vi "Draw Object Tree.vi"() -> ()   [LabVIEW 2019]
uses:
  Logger_class/ObjData.ctl
  Logger_class/ObjType.ctl
  Logger_class/Logger.lvclass
panel:
  out "All Objects":set{T1}(c389)={{"object_tag"="AI0", "parent_tag"="STAND", "object_type"=enum."AI", "description"="Óðîâåíü  ìàñëà"}, {"object_tag"="AI0.HI", "parent_tag"="AI0", "object_type"=enum."AA", "description"="AI0.HI"}, {"object_tag"="AI0.HIHI", "parent_tag"="AI0", "object_type"=enum."AA", "description"="AI0.HIHI"}, {"object_tag"="AI0.LO", "parent_tag"="AI0", "object_type"=enum."AA", "description"="AI0.LO"}, {"object_tag"="AI0.LOLO", "parent_tag"="AI0", "object_type"=enum."AA", "description"="AI0.LOLO"}, {"object_tag"="AI0.OutOfRangeMax", "parent_tag"="AI0", "object_type"=enum."AA", "description"="AI0.OutOfRangeMax"}, {"object_tag"="AI0.OutOfRangeMin", "parent_tag"="AI0", "object_type"=enum."AA", "description"="AI0.OutOfRangeMin"}, {"object_tag"="AI1", "parent_tag"="STAND", "object_type"=enum."AI", "description"="Óðîâåíü  ìàñëà"}, {"object_tag"="AI1.HI", "parent_tag"="AI1", "object_type"=enum."AA", "description"="AI1.HI"}, {"object_tag"="AI1.HIHI", "parent_tag"="AI1", "object_type"=enum."AA", "description"="AI1.HIHI"}, {"object_tag"="AI1.LO", "parent_tag"="AI1", "object_type"=enum."AA", "description"="AI1.LO"}, {"object_tag"="AI1.LOLO", "parent_tag"="AI1", "object_type"=enum."AA", "description"="AI1.LOLO"}, {"object_tag"="AI1.OutOfRangeMax", "parent_tag"="AI1", "object_type"=enum."AA", "description"="AI1.OutOfRangeMax"}, {"object_tag"="AI1.OutOfRangeMin", "parent_tag"="AI1", "object_type"=enum."AA", "description"="AI1.OutOfRangeMin"}, {"object_tag"="AI10", "parent_tag"="STAND", "object_type"=enum."AI", "description"="Äàò÷èê äàâëåíèÿ â ëèíèè èçìåðåíèÿ óòå÷åê"}, {"object_tag"="AI10.HI", "parent_tag"="AI10", "object_type"=enum."AA", "description"="AI10.HI"}, {"object_tag"="AI10.HIHI", "parent_tag"="AI10", "object_type"=enum."AA", "description"="AI10.HIHI"}, {"object_tag"="AI10.LO", "parent_tag"="AI10", "object_type"=enum."AA", "description"="AI10.LO"}, {"object_tag"="AI10.LOLO", "parent_tag"="AI10", "object_type"=enum."AA", "description"="AI10.LOLO"}, {"object_tag"="AI10.OutOfRangeMax", "parent_tag"="AI10", "object_type"=enum."AA", "description"="AI10.OutOfRangeMax"}, {"object_tag"="AI10.OutOfRangeMin", "parent_tag"="AI10", "object_type"=enum."AA", "description"="AI10.OutOfRangeMin"}, {"object_tag"="AI2", "parent_tag"="STAND", "object_type"=enum."AI", "description"="Òåìïåðàòóðà ìàñëà"}, {"object_tag"="AI2.HI", "parent_tag"="AI2", "object_type"=enum."AA", "description"="AI2.HI"}, {"object_tag"="AI2.HIHI", "parent_tag"="AI2", "object_type"=enum."AA", "description"="AI2.HIHI"}, {"object_tag"="AI2.LO", "parent_tag"="AI2", "object_type"=enum."AA", "description"="AI2.LO"}, {"object_tag"="AI2.LOLO", "parent_tag"="AI2", "object_type"=enum."AA", "description"="AI2.LOLO"}, {"object_tag"="AI2.OutOfRangeMax", "parent_tag"="AI2", "object_type"=enum."AA", "description"="AI2.OutOfRangeMax"}, {"object_tag"="AI2.OutOfRangeMin", "parent_tag"="AI2", "object_type"=enum."AA", "description"="AI2.OutOfRangeMin"}, {"object_tag"="AI3", "parent_tag"="STAND", "object_type"=enum."AI", "description"="Òåìïåðàòóðà ìàñëà"}, {"object_tag"="AI3.HI", "parent_tag"="AI3", "object_type"=enum."AA", "description"="AI3.HI"}, {"object_tag"="AI3.HIHI", "parent_tag"="AI3", "object_type"=enum."AA", "description"="AI3.HIHI"}, {"object_tag"="AI3.LO", "parent_tag"="AI3", "object_type"=enum."AA", "description"="AI3.LO"}, {"object_tag"="AI3.LOLO", "parent_tag"="AI3", "object_type"=enum."AA", "description"="AI3.LOLO"}, {"object_tag"="AI3.OutOfRangeMax", "parent_tag"="AI3", "object_type"=enum."AA", "description"="AI3.OutOfRangeMax"}, {"object_tag"="AI3.OutOfRangeMin", "parent_tag"="AI3", "object_type"=enum."AA", "description"="AI3.OutOfRangeMin"}, {"object_tag"="AI4", "parent_tag"="STAND", "object_type"=enum."AI", "description"="Îáðàòíàÿ ñâÿçü  îò êëàïàíà"}, {"object_tag"="AI4.HI", "parent_tag"="AI4", "object_type"=enum."AA", "description"="AI4.HI"}, {"object_tag"="AI4.HIHI", "parent_tag"="AI4", "object_type"=enum."AA", "description"="AI4.HIHI"}, {"object_tag"="AI4.LO", "parent_tag"="AI4", "object_type"=enum."AA", "description"="AI4.LO"}, {"object_tag"="AI4.LOLO", "parent_tag"="AI4", "object_type"=enum."AA", "description"="AI4.LOLO"}, {"object_tag"="AI4.OutOfRangeMax", "parent_tag"="AI4", "object_type"=enum."AA", "description"="AI4.OutOfRangeMax"}, {"object_tag"="AI4.OutOfRangeMin", "parent_tag"="AI4", "object_type"=enum."AA", "description"="AI4.OutOfRangeMin"}, {"object_tag"="AI5", "parent_tag"="STAND", "object_type"=enum."AI", "description"="äàâëåíèå ïîñëå íàñîñà ÂÄ"}, {"object_tag"="AI5.HI", "parent_tag"="AI5", "object_type"=enum."AA", "description"="AI5.HI"}, {"object_tag"="AI5.HIHI", "parent_tag"="AI5", "object_type"=enum."AA", "description"="AI5.HIHI"}, {"object_tag"="AI5.LO", "parent_tag"="AI5", "object_type"=enum."AA", "description"="AI5.LO"}, {"object_tag"="AI5.LOLO", "parent_tag"="AI5", "object_type"=enum."AA", "description"="AI5.LOLO"}, {"object_tag"="AI5.OutOfRangeMax", "parent_tag"="AI5", "object_type"=enum."AA", "description"="AI5.OutOfRangeMax"}, {"object_tag"="AI5.OutOfRangeMin", "parent_tag"="AI5", "object_type"=enum."AA", "description"="AI5.OutOfRangeMin"}, {"object_tag"="AI6", "parent_tag"="STAND", "object_type"=enum."AI", "description"="Äàâëåíèå â îáðàçöå"}, {"object_tag"="AI6.HI", "parent_tag"="AI6", "object_type"=enum."AA", "description"="AI6.HI"}, {"object_tag"="AI6.HIHI", "parent_tag"="AI6", "object_type"=enum."AA", "description"="AI6.HIHI"}, {"object_tag"="AI6.LO", "parent_tag"="AI6", "object_type"=enum."AA", "description"="AI6.LO"}, {"object_tag"="AI6.LOLO", "parent_tag"="AI6", "object_type"=enum."AA", "description"="AI6.LOLO"}, {"object_tag"="AI6.OutOfRangeMax", "parent_tag"="AI6", "object_type"=enum."AA", "description"="AI6.OutOfRangeMax"}, {"object_tag"="AI6.OutOfRangeMin", "parent_tag"="AI6", "object_type"=enum."AA", "description"="AI6.OutOfRangeMin"}, {"object_tag"="AI7", "parent_tag"="STAND", "object_type"=enum."AI", "description"="Äàâëåíèå â êàìåðå"}, {"object_tag"="AI7.HI", "parent_tag"="AI7", "object_type"=enum."AA", "description"="AI7.HI"}, {"object_tag"="AI7.HIHI", "parent_tag"="AI7", "object_type"=enum."AA", "description"="AI7.HIHI"}, {"object_tag"="AI7.LO", "parent_tag"="AI7", "object_type"=enum."AA", "description"="AI7.LO"}, {"object_tag"="AI7.LOLO", "parent_tag"="AI7", "object_type"=enum."AA", "description"="AI7.LOLO"}, {"object_tag"="AI7.OutOfRangeMax", "parent_tag"="AI7", "object_type"=enum."AA", "description"="AI7.OutOfRangeMax"}, {"object_tag"="AI7.OutOfRangeMin", "parent_tag"="AI7", "object_type"=enum."AA", "description"="AI7.OutOfRangeMin"}, {"object_tag"="AI8", "parent_tag"="STAND", "object_type"=enum."AI", "description"="Äàâëåíèå  â  ëèíèè ïîäà÷è âîçäóõà â  áëîê ÏÏÂ"}, {"object_tag"="AI8.HI", "parent_tag"="AI8", "object_type"=enum."AA", "description"="AI8.HI"}, {"object_tag"="AI8.HIHI", "parent_tag"="AI8", "object_type"=enum."AA", "description"="AI8.HIHI"}, {"object_tag"="AI8.LO", "parent_tag"="AI8", "object_type"=enum."AA", "description"="AI8.LO"}, {"object_tag"="AI8.LOLO", "parent_tag"="AI8", "object_type"=enum."AA", "description"="AI8.LOLO"}, {"object_tag"="AI8.OutOfRangeMax", "parent_tag"="AI8", "object_type"=enum."AA", "description"="AI8.OutOfRangeMax"}, {"object_tag"="AI8.OutOfRangeMin", "parent_tag"="AI8", "object_type"=enum."AA", "description"="AI8.OutOfRangeMin"}, {"object_tag"="AI9", "parent_tag"="STAND", "object_type"=enum."AI", "description"="Äàâëåíèå  â  ëèíèè ïîäà÷è âîçäóõà ïîñëå áëîêà ÏÏÂ"}, {"object_tag"="AI9.HI", "parent_tag"="AI9", "object_type"=enum."AA", "description"="AI9.HI"}, {"object_tag"="AI9.HIHI", "parent_tag"="AI9", "object_type"=enum."AA", "description"="AI9.HIHI"}, {"object_tag"="AI9.LO", "parent_tag"="AI9", "object_type"=enum."AA", "description"="AI9.LO"}, {"object_tag"="AI9.LOLO", "parent_tag"="AI9", "object_type"=enum."AA", "description"="AI9.LOLO"}, {"object_tag"="AI9.OutOfRangeMax", "parent_tag"="AI9", "object_type"=enum."AA", "description"="AI9.OutOfRangeMax"}, {"object_tag"="AI9.OutOfRangeMin", "parent_tag"="AI9", "object_type"=enum."AA", "description"="AI9.OutOfRangeMin"}, {"object_tag"="DI0", "parent_tag"="STAND", "object_type"=enum."DI", "description"="Êîíòàêòîð"}, {"object_tag"="DI1", "parent_tag"="STAND", "object_type"=enum."DI", "description"="Àâòîìàò"}, {"object_tag"="DI10", "parent_tag"="STAND", "object_type"=enum."DI", "description"="QF4"}, {"object_tag"="DI11", "parent_tag"="STAND", "object_type"=enum."DI", "description"="QF5"}, {"object_tag"="DI12", "parent_tag"="STAND", "object_type"=enum."DI", "description"="Êíîïêà ñáðîñà îøèáêè SB1"}, {"object_tag"="DI13", "parent_tag"="STAND", "object_type"=enum."DI", "description"="Êíîïêà çàïóñêà SB2"}, {"object_tag"="DI14", "parent_tag"="STAND", "object_type"=enum."DI", "description"="Êíîïêà îñòàíîâêè SB3"}, {"object_tag"="DI15", "parent_tag"="STAND", "object_type"=enum."DI", "description"="Êíîïêà àâàðèéíîé îñòàíîâêè SB4"}, {"object_tag"="DI16", "parent_tag"="STAND", "object_type"=enum."DI", "description"="Ïåðåêëþ÷àòåëü ðó÷íîå/àâòî SA1"}, {"object_tag"="DI17", "parent_tag"="STAND", "object_type"=enum."DI", "description"="Èñòî÷íèê ïèòàíèÿ 24 Â"}, {"object_tag"="DI18", "parent_tag"="STAND", "object_type"=enum."DI", "description"="DI 18"}, {"object_tag"="DI19", "parent_tag"="STAND", "object_type"=enum."DI", "description"="DI 19"}, {"object_tag"="DI2", "parent_tag"="STAND", "object_type"=enum."DI", "description"="Êîíòàêòîð"}, {"object_tag"="DI20", "parent_tag"="STAND", "object_type"=enum."DI", "description"="DI 20"}, {"object_tag"="DI21", "parent_tag"="STAND", "object_type"=enum."DI", "description"="DI 21"}, {"object_tag"="DI22", "parent_tag"="STAND", "object_type"=enum."DI", "description"="DI 22"}, {"object_tag"="DI23", "parent_tag"="STAND", "object_type"=enum."DI", "description"="DI 23"}, {"object_tag"="DI24", "parent_tag"="STAND", "object_type"=enum."DI", "description"="DI 24"}, {"object_tag"="DI25", "parent_tag"="STAND", "object_type"=enum."DI", "description"="DI 25"}, {"object_tag"="DI26", "parent_tag"="STAND", "object_type"=enum."DI", "description"="DI 26"}, {"object_tag"="DI27", "parent_tag"="STAND", "object_type"=enum."DI", "description"="DI 27"}, {"object_tag"="DI28", "parent_tag"="STAND", "object_type"=enum."DI", "description"="DI 28"}, {"object_tag"="DI29", "parent_tag"="STAND", "object_type"=enum."DI", "description"="DI 29"}, {"object_tag"="DI3", "parent_tag"="STAND", "object_type"=enum."DI", "description"="Àâòîìàò"}, {"object_tag"="DI30", "parent_tag"="STAND", "object_type"=enum."DI", "description"="DI 30"}, {"object_tag"="DI31", "parent_tag"="STAND", "object_type"=enum."DI", "description"="DI 31"}, {"object_tag"="DI4", "parent_tag"="STAND", "object_type"=enum."DI", "description"="Êîíòàêòîð"}, {"object_tag"="DI5", "parent_tag"="STAND", "object_type"=enum."DI", "description"="Àâòîìàò"}, {"object_tag"="DI6", "parent_tag"="STAND", "object_type"=enum."DI", "description"="QF1"}, {"object_tag"="DI7", "parent_tag"="STAND", "object_type"=enum."DI", "description"="QF2"}, {"object_tag"="DI8", "parent_tag"="STAND", "object_type"=enum."DI", "description"="QF3"}, {"object_tag"="DI9", "parent_tag"="STAND", "object_type"=enum."DI", "description"="Ðåëå êîíòðîëÿ ôàç"}, {"object_tag"="M12", "parent_tag"="PMG", "object_type"=enum."Device", "description"="M12"}, {"object_tag"="M12.Contactor Error", "parent_tag"="M12", "object_type"=enum."DA", "description"=""}, {"object_tag"="M12.OFF_Error", "parent_tag"="M12", "object_type"=enum."DA", "description"=""}, {"object_tag"="M12.ON_Error", "parent_tag"="M12", "object_type"=enum."DA", "description"=""}, {"object_tag"="M12.UnOFF_Error", "parent_tag"="M12", "object_type"=enum."DA", "description"=""}, {"object_tag"="M12.UnON_Error", "parent_tag"="M12", "object_type"=enum."DA", "description"=""}, {"object_tag"="M21", "parent_tag"="PMG", "object_type"=enum."Device", "description"="M21"}, {"object_tag"="M21.Contactor Error", "parent_tag"="M21", "object_type"=enum."DA", "description"=""}, {"object_tag"="M21.OFF_Error", "parent_tag"="M21", "object_type"=enum."DA", "description"=""}, {"object_tag"="M21.ON_Error", "parent_tag"="M21", "object_type"=enum."DA", "description"=""}, {"object_tag"="M21.UnOFF_Error", "parent_tag"="M21", "object_type"=enum."DA", "description"=""}, {"object_tag"="M21.UnON_Error", "parent_tag"="M21", "object_type"=enum."DA", "description"=""}, {"object_tag"="M22", "parent_tag"="PMG", "object_type"=enum."Device", "description"="M22"}, {"object_tag"="M22.Contactor Error", "parent_tag"="M22", "object_type"=enum."DA", "description"=""}, {"object_tag"="M22.OFF_Error", "parent_tag"="M22", "object_type"=enum."DA", "description"=""}, {"object_tag"="M22.ON_Error", "parent_tag"="M22", "object_type"=enum."DA", "description"=""}, {"object_tag"="M22.UnOFF_Error", "parent_tag"="M22", "object_type"=enum."DA", "description"=""}, {"object_tag"="M22.UnON_Error", "parent_tag"="M22", "object_type"=enum."DA", "description"=""}, {"object_tag"="NV1", "parent_tag"="STAND", "object_type"=enum."Device", "description"="NV1"}, {"object_tag"="NV2", "parent_tag"="STAND", "object_type"=enum."Device", "description"="NV2"}, {"object_tag"="PMG", "parent_tag"="STAND", "object_type"=enum."Device", "description"="PMG"}, {"object_tag"="STAND", "parent_tag"="", "object_type"=enum."Device", "description"=""}, {"object_tag"="VALVE_44_1", "parent_tag"="STAND", "object_type"=enum."Device", "description"="VALVE_44_1"}, {"object_tag"="VALVE_44_2", "parent_tag"="STAND", "object_type"=enum."Device", "description"="VALVE_44_2"}}
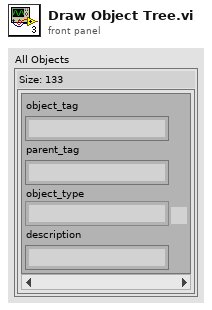
[diagram p1: front panel]
types:
  T1 = typedef "Logger.lvclass/ObjData.ctl" = cluster{"object_tag":string, "parent_tag":string, "object_type":T2, "description":string}
  T2 = typedef "Logger.lvclass/ObjType.ctl" = enum16{"Procces", "Device", "Signal", "DI", "DO", "DA", "AI", "AO", "AA"}
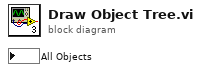
[diagram p0: block diagram]
diagram:
